vi "Grid Measurements Example - Potential.vi"(6 "Internal use":string, 7 "Grid param":T1 {"height (m)" format="%#_6p"; "width (m)" format="%#_6p"; "center Y (m)" format="%#_6p"; "center X (m)" format="%#_6p"}, 8 "Error in (no error)":errorcluster, 9 "Points Y/Index Y":i32, 10 "Points X/Index X":i32, 11 "Method":enum16{"init", "run", "end"}(ring)) -> (0 "Error out":errorcluster)   [LabVIEW 2017]
doc: "Example of a measurement VI to be used in the \"Experiments on a Grid\" tool as external VI.\n\nThis example measures a potential difference map by performing bias spectroscopy and fitting a parabola to the Frequency Shift.\n\n- Nanonis Programming Interface -"
uses:
  Nanonis Prog Interface.lvlib
  <vilib>/Analysis/NI_AALPro.lvlib
  Instance           1 45Saved   Grid Measurements Example - Potential .vi
panel:
  # "Example of a measurement VI to be used in the \"Experiments on a Grid\" tool as external VI.\n\nThis example measure a potential difference map.\n\nTo use it, set up the bias spectroscopy module to record the \"Frequency shift\" and set all other parameters to the desired value. Then, set up the \"experiments on a grid\" module to use this VI as \"external VI\".\n\n\"Experiments on a Grid\" will first (before starting the measurements) call the external VI with the \"init\" method, passing the grid resolution (Points X, Points Y) and the grid dimensions (Grid param).\nThen, for the measurements, the external VI will be called with the \"run\" method, passing the current X and Y indices (Index X, Index Y).\nAfter the last measurement, the external VI will be called with the \"end\" method.\n\nSee diagram for more information about this example."
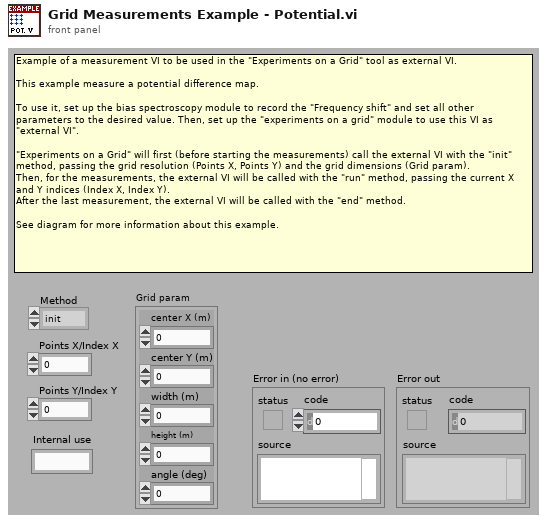
[diagram p1: front panel]
types:
  T1 = cluster{"center X (m)":sgl, "center Y (m)":sgl, "width (m)":sgl, "height (m)":sgl, "angle (deg)":sgl}
  T2 = cluster{"Name":string, "Calibration":sgl, "Offset":sgl, "Channel index":i32}[]
  T3 = cluster{"center X":sgl, "center Y":sgl, "angle":sgl, "width":sgl, "height":sgl, "# pixels":i32, "# lines":i32}
  T4 = cluster{"up/down":bool, "time/line":sgl, "start time":timestamp, "end time":timestamp}
  T5 = enum32{"SVD", "Givens", "Givens2", "Householder", "LU Decomposition", "Cholesky"}
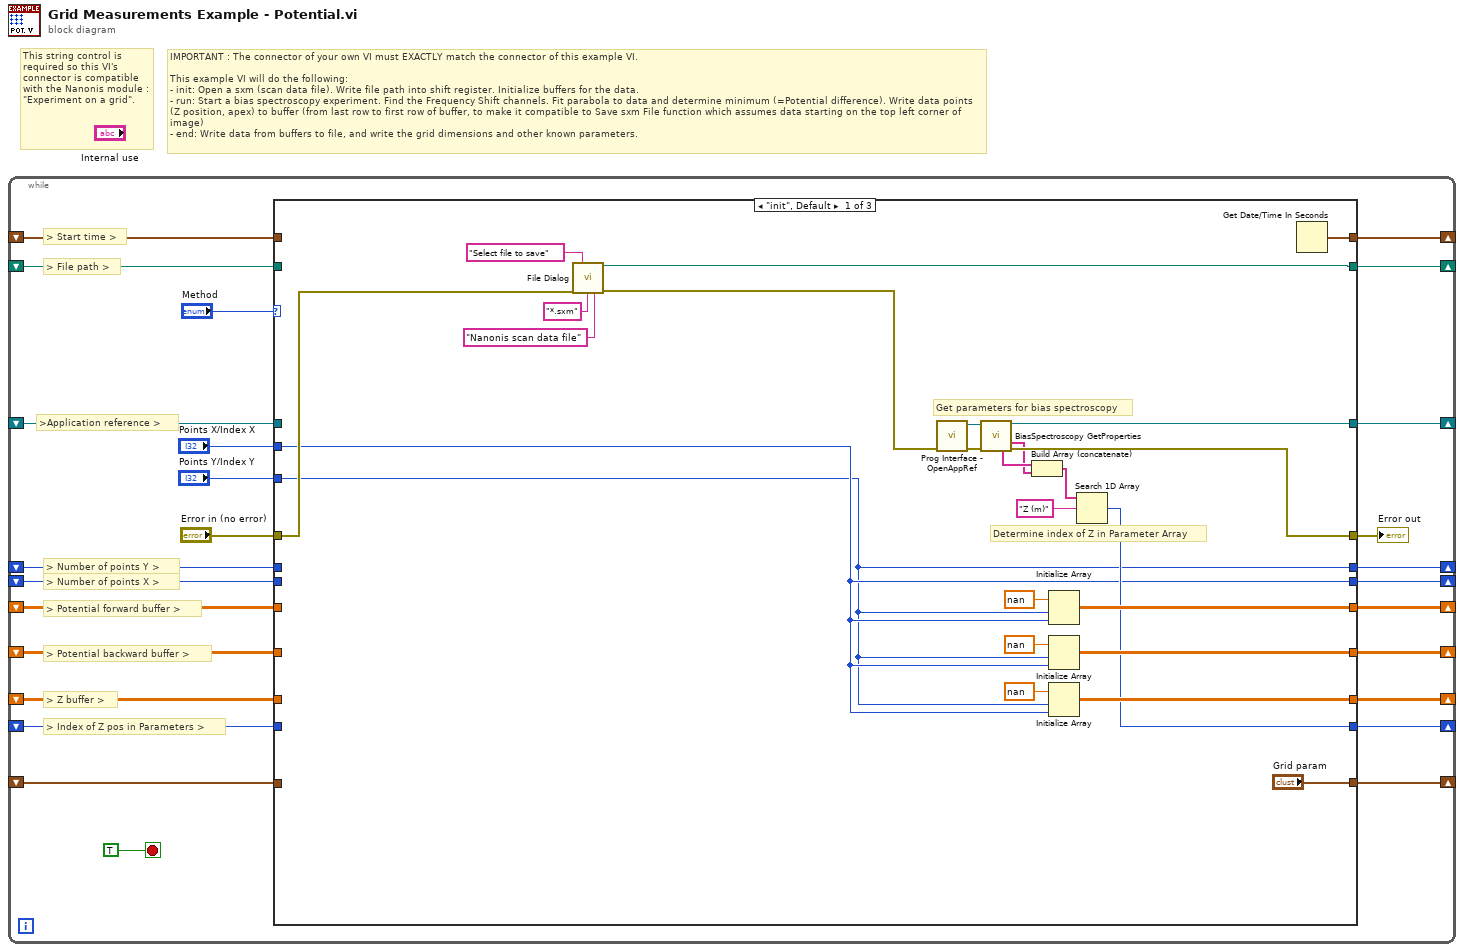
[diagram p0: block diagram]
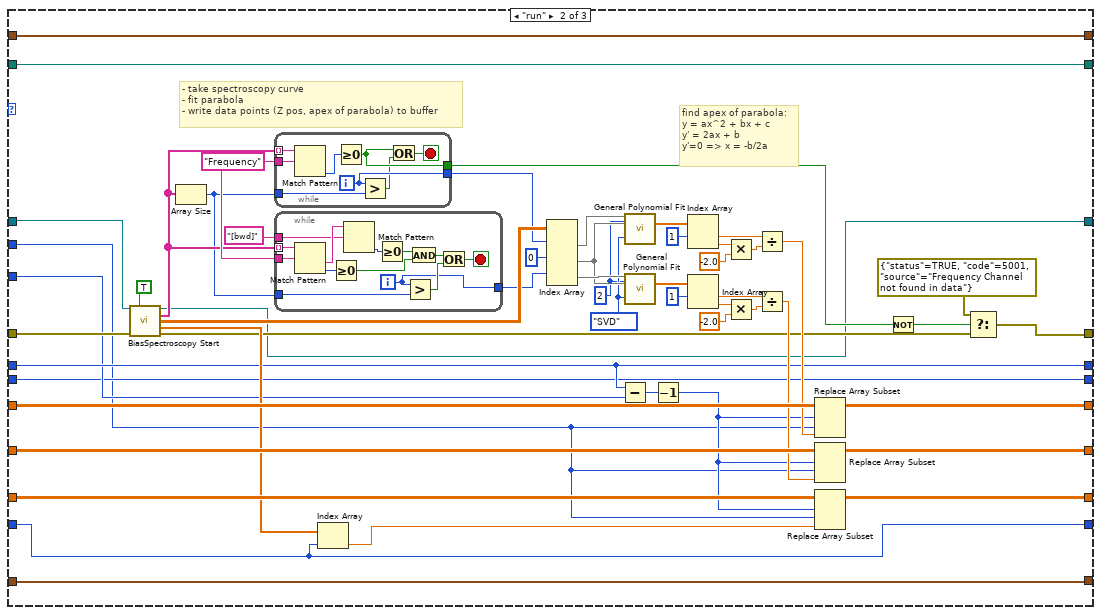
[diagram p2: hidden frame]
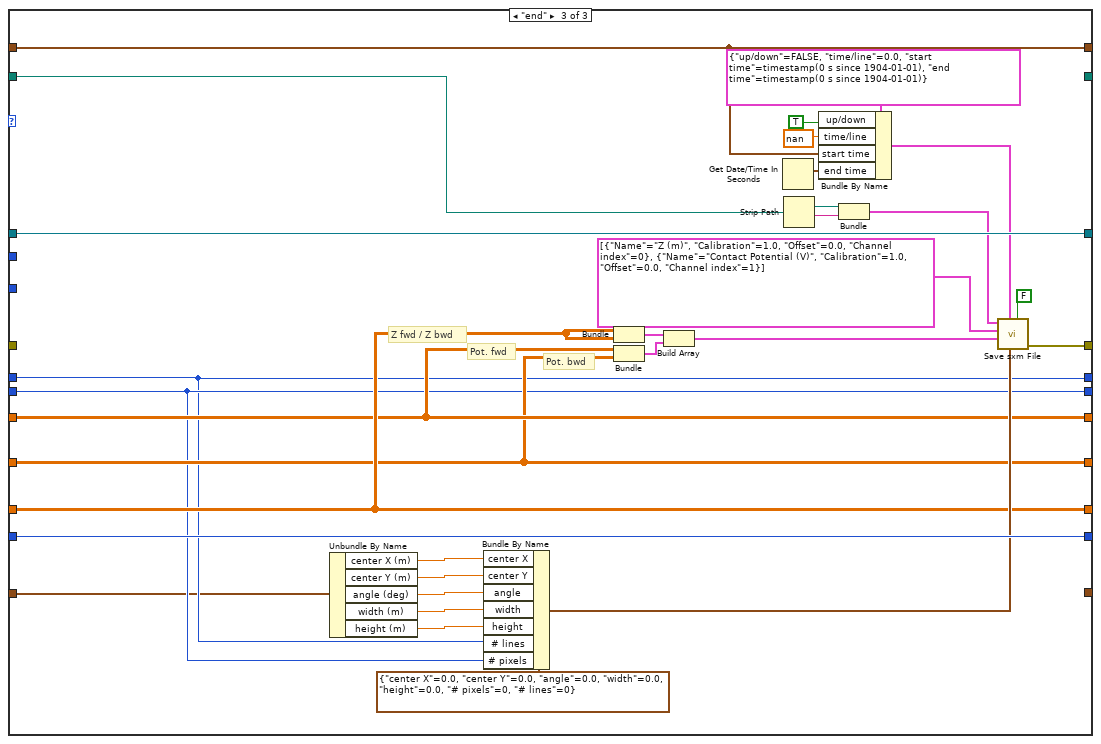
[diagram p3: hidden frame]
diagram:
  # "This string control is required so this VI's connector is compatible with the Nanonis module : \"Experiment on a grid\"."
  # "IMPORTANT : The connector of your own VI must EXACTLY match the connector of this example VI.\n\nThis example VI will do the following:\n- init: Open a sxm (scan data file). Write file path into shift register. Initialize buffers for the data.\n- run: Start a bias spectroscopy experiment. Find the Frequency Shift channels. Fit parabola to data and determine minimum (=Potential difference). Write data points (Z position, apex) to buffer (from last row to first row of buffer, to make it compatible to Save sxm File function which assumes data starting on the top left corner of image)\n- end: Write data from buffers to file, and write the grid dimensions and other known parameters."
  n1 = while {
    shift-right: [w24] -> _
    shift-left: _ -> [w23]
    shift-right: [w18] -> _
    shift-left: _ -> [w17]
    shift-right: [w16] -> _
    shift-left: _ -> [w15]
    shift-right: [w14] -> _
    shift-left: _ -> [w13]
    shift-right: [w12] -> _
    shift-left: _ -> [w11]
    shift-right: [w10] -> _
    shift-left: _ -> [w9]
    shift-right: [w8] -> _
    shift-left: _ -> [w7]
    shift-right: [w6] -> _
    shift-left: _ -> [w5]
    shift-right: [w4] -> _
    shift-left: _ -> [w3]
    shift-right: [w2] -> _
    shift-left: _ -> [w1]
    stop <- TRUE stop-if-true
    # "> Number of points Y >"
    # "> Start time >"
    # ">Application reference >"
    # "> Index of Z pos in Parameters >"
    # "> Z buffer >"
    # "> Potential backward buffer >"
    # "> Potential forward buffer >"
    # "> Number of points X >"
    # "> File path >"
    n2 = case shown="\"init\", Default" "Method" {
      tunnel: [w31 w99 _] -> w24
      tunnel: w23 -> [_ w99 w144]
      tunnel: "Error in (no error)" -> [w33 w105 _]
      tunnel: [w45 w67 w151] -> w21
      tunnel: "Points X/Index X" -> [w29 w53 _]
      tunnel: "Points Y/Index Y" -> [w28 w57 _]
      tunnel: [w50 w100 w131] -> w18
      tunnel: w17 -> [_ w101 w131]
      tunnel: [w48 w97 w130] -> w16
      tunnel: w15 -> [_ w96 w130]
      tunnel: [w29 w54 w129] -> w14
      tunnel: w13 -> [_ w54 w129]
      tunnel: [w47 w88 w132] -> w12
      tunnel: w11 -> [_ w89 w132]
      tunnel: [w43 w73 w157] -> w10
      tunnel: w9 -> [_ w73 w157]
      tunnel: [w37 w61 w156] -> w8
      tunnel: w7 -> [_ w62 w156]
      tunnel: [w30 w59 w149] -> w6
      tunnel: w5 -> [_ w59 w149]
      tunnel: [w28 w58 w128] -> w4
      tunnel: w3 -> [_ w58 w128]
      tunnel: w1 -> [_ w52 w127]
      tunnel: ["Grid param" w52 _] -> w2
      frame "init", Default {
        # "Get parameters for bias spectroscopy"
        # "Determine index of Z in Parameter Array"
        n3 = call "File Dialog"("prompt"="Select file to save", "error in"=w33, "pattern (all files)"="*.sxm" ("pattern"), "pattern label"="Nanonis scan data file") -> ("selected path"=w31:path, "error out"=w32:errorcluster)  [unwired: 8 in, 2 out]
        n4 = call <userlib>:"Prog Interface - OpenAppRef.vi"("Error in (no error)"=w32) -> ("Error out"=w39:errorcluster, "Application reference"=w38:refnum<vi>)  [unwired: 5 in]
        n5 = call <userlib>:"BiasSpectroscopy GetProperties.vi"("Application ref in"=w38, "Error in (no error)"=w39) -> ("Application ref out"=w37:refnum<vi>, "Parameters"=w41:string[], "Fixed parameters"=w42:string[], "Error out"=w45:errorcluster)  [unwired: 6 in, 4 out]
        n6 = Build Array (concatenate)(w42, w41) -> (w40:string[])
        n7 = Initialize Array(sgl nan ("element"), w28, w29) -> (w50:sgl[][])
        n8 = Initialize Array(sgl nan ("element"), w28, w29) -> (w48:sgl[][])
        n9 = Initialize Array(sgl nan ("element"), w28, w29) -> (w47:sgl[][])
        n10 = Search 1D Array(1D array=w40, element="Z (m)") -> (index of element=w43:i32)  [unwired: 1 in]
        n11 = Get Date/Time In Seconds() -> (seconds since 1Jan1904=w30:timestamp)
      }
      frame "run" {
        w70 = T5."SVD" ("algorithm")
        w69 = 2 ("polynomial order")
        w95 = "Frequency"
        # "find apex of parabola:\ny = ax^2 + bx + c\ny' = 2ax + b\ny'=0 => x = -b/2a"
        # "- take spectroscopy curve\n- fit parabola\n- write data points (Z pos, apex of parabola) to buffer"
        n12 = call <userlib>:"BiasSpectroscopy Start.vi"("Application ref in"=w62, "Get data (F)"=TRUE ("Get Data (F)"), "Error in (no error)"=w105) -> ("Application ref out"=w61:refnum<vi>, "Channels"=w72:string[], "Data"=w104:sgl[][], "Parameters"=w66:sgl[], "Error out"=w64:errorcluster)  [unwired: 8 in]
        n13 = Array Size(array=w72) -> (size(s)=w71:i32)
        n14 = while {
          tunnel: w72 -> [w126] mode=indexing
          tunnel: w95 -> [w125]
          tunnel: [w122] -> w98
          tunnel: w71 -> [w123]
          tunnel: [w121] -> w68
          i -> [w122]
          stop <- w120 stop-if-true
          n15 = Match Pattern(string=w126, regular expression=w125) -> (offset past match=w124:i32)  [unwired: 1 in, 3 out]
          n16 = Greater Or Equal To 0?(x=w124) -> (x >= 0?=w121:bool)
          n17 = Greater?(x=w122, y=w123) -> (0:w119:bool)
          n18 = Or(x=w121, y=w119) -> (x .or. y?=w120:bool)
        }
        n19 = while {
          tunnel: w72 -> [w118] mode=indexing
          tunnel: w95 -> [w117]
          tunnel: [w107] -> w93
          tunnel: "[bwd]" ("regular expression") -> [w114]
          tunnel: w71 -> [w110]
          i -> [w107]
          stop <- w108 stop-if-true
          n20 = Match Pattern(string=w118, regular expression=w117) -> (after substring=w115:string, offset past match=w116:i32)  [unwired: 1 in, 2 out]
          n21 = Greater Or Equal To 0?(x=w116) -> (x >= 0?=w112:bool)
          n22 = Match Pattern(string=w115, regular expression=w114) -> (offset past match=w113:i32)  [unwired: 1 in, 3 out]
          n23 = Greater Or Equal To 0?(x=w113) -> (x >= 0?=w111:bool)
          n24 = Greater?(x=w107, y=w110) -> (0:w109:bool)
          n25 = And(x=w111, y=w112) -> (x .and. y?=w106:bool)
          n26 = Or(x=w106, y=w109) -> (x .or. y?=w108:bool)
        }
        n27 = Index Array(array=w66, index=w73) -> (element=w74:sgl)
        n28 = Index Array(array=w104, index (row) #1=w98, index (row) #2=0 ("index (row)"), index (row) #3=w93) -> (element #1=w75:sgl[], element #2=w76:sgl[], element #3=w90:sgl[])  [unwired: 3 in]
        n29 = Subtract(x=w58, y=w57) -> (x-y=w56:i32)
        n30 = call <vilib>:"General Polynomial Fit.vi"("Y"=w75, "polynomial order"=w69, "X"=w76, "algorithm"=w70) -> ("Polynomial Coefficients"=w85:dbl[])  [unwired: 8 in, 3 out]
        n31 = call <vilib>:"General Polynomial Fit.vi"("Y"=w90, "polynomial order"=w69, "X"=w76, "algorithm"=w70) -> ("Polynomial Coefficients"=w91:dbl[])  [unwired: 8 in, 3 out]
        n32 = Decrement(x=w56) -> (x-1=w55:i32)
        n33 = Index Array(array=w85, index #1=1 ("index")) -> (element #1=w83:dbl, element #2=w84:dbl)  [unwired: 1 in]
        n34 = Index Array(array=w91, index #1=1 ("index")) -> (element #1=w78:dbl, element #2=w79:dbl)  [unwired: 1 in]
        n35 = Multiply(x=w84, y=-2.0) -> (x*y=w86:dbl)
        n36 = Multiply(x=w79, y=-2.0) -> (x*y=w81:dbl)
        n37 = Divide(x=w83, y=w86) -> (x/y=w82:dbl)
        n38 = Divide(x=w78, y=w81) -> (x/y=w77:dbl)
        n39 = Replace Array Subset(array=w101, new element=w82, index (row)=w55, index (col)=w53) -> (w100:sgl[][])
        n40 = Replace Array Subset(array=w96, new element=w77, index (row)=w55, index (col)=w53) -> (w97:sgl[][])
        n41 = Replace Array Subset(array=w89, new element=w74, index (row)=w55, index (col)=w53) -> (w88:sgl[][])
        n42 = Not(x=w68) -> (.not. x?=w65:bool)
        n43 = Select(t=errorcluster {"status"=TRUE, "code"=5001, "source"="Frequency Channel not found in data"} ("f"), s=w65, f=w64) -> (s? t:f=w67:errorcluster)
      }
      frame "end" {
        # "Pot. bwd"
        # "Pot. fwd"
        # "Z fwd / Z bwd"
        n44 = Unbundle By Name(w127) -> ("center X (m)"=w139:sgl, "center Y (m)"=w140:sgl, "angle (deg)"=w141:sgl, "width (m)"=w142:sgl, "height (m)"=w143:sgl)
        n45 = Bundle By Name(cluster=T3 {"center X"=0.0, "center Y"=0.0, "angle"=0.0, "width"=0.0, "height"=0.0, "# pixels"=0, "# lines"=0} ("Scanfield"), "center X"=w139, "center Y"=w140, "angle"=w141, "width"=w142, "height"=w143, "# lines"=w128, "# pixels"=w129) -> (w137:T3)
        n46 = Bundle(w132, w132) -> (w135:cluster{sgl[][], sgl[][]})  [unwired: 1 in]
        n47 = Bundle(w131, w130) -> (w133:cluster{sgl[][], sgl[][]})  [unwired: 1 in]
        n48 = Build Array(w135, w133) -> (w134:cluster{sgl[][], sgl[][]}[])
        n49 = Get Date/Time In Seconds() -> (seconds since 1Jan1904=w153:timestamp)
        n50 = Strip Path(path=w144) -> (stripped path=w148:path, name=w147:string)
        n51 = Bundle By Name(cluster=T4 {"up/down"=FALSE, "time/line"=0.0, "start time"=timestamp(0 s since 1904-01-01), "end time"=timestamp(0 s since 1904-01-01)} ("Scan param"), "up/down"=TRUE, "time/line"=sgl nan ("input 7"), "start time"=w149, "end time"=w153) -> (w150:T4)
        n52 = Bundle("stripped path"=w148, "name"=w147) -> (w145:cluster{"stripped path":path, "name":string})  [unwired: 1 in]
        n53 = call "Save sxm File.vi"("Auto file naming? (T)"=FALSE, "Scanfield"=w137, "Scan param"=w150, "Channels data"=w134, "Channels config"=T2 [{"Name"="Z (m)", "Calibration"=1.0, "Offset"=0.0, "Channel index"=0}, {"Name"="Contact Potential (V)", "Calibration"=1.0, "Offset"=0.0, "Channel index"=1}], "Filename control"=w145) -> ("error out"=w151:errorcluster)  [unwired: 3 in, 2 out]
      }
    }
    "Error out" <- w21
  }
